vi "Find MFStruct Inner Tunnel.vi"(7 "Source? (T)":bool=TRUE, 8 "error in (no error)":errorcluster, 9 "Tunnel Name":string, 10 "Contained GObject":refnum<vi>, 11 "MFStruct":refnum<vi>) -> (0 "error IO":errorcluster, 1 "Inside Tunnel":refnum<vi>, 2 "GObject dup":refnum<vi>, 3 "MFStruct dup":refnum<vi>)   [LabVIEW 2022 SP3, in "FlexBlocks Support.lvlib"]
uses:
  FlexBlocks Support.lvlib
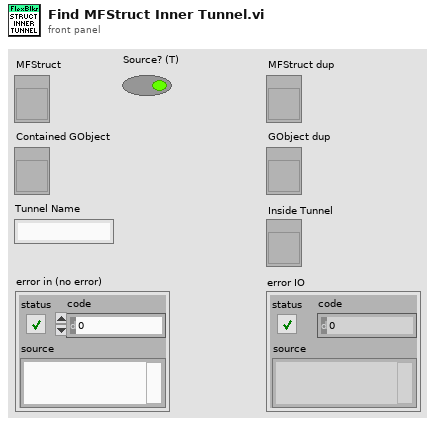
[diagram p1: front panel]
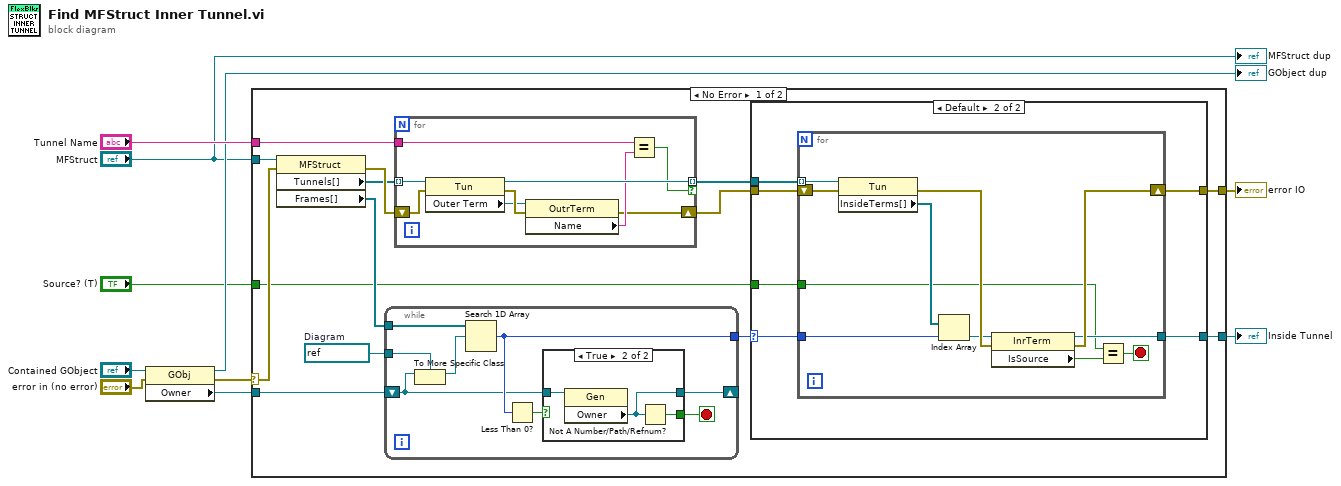
[diagram p0: block diagram]
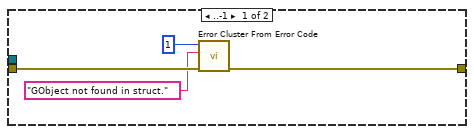
[diagram p2: hidden frame]
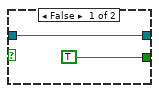
[diagram p3: hidden frame]
diagram:
  n1 = property class="GObj"(reference="Contained GObject", error in="error in (no error)") -> (reference out=→"GObject dup":refnum<vi>, error out=w5:errorcluster, "Owner"=w4:refnum<vi>)
  n2 = case shown="No Error" w5 {
    selector: w5 -> [w20 w68]
    tunnel: "MFStruct" -> [w23 _]
    tunnel: w4 -> [w22 _]
    tunnel: "Tunnel Name" -> [w18 _]
    tunnel: [w16 w68] -> w7
    tunnel: [w13 _] -> w8
    tunnel: "Source? (T)" -> [w11 _]
    frame No Error {
      w12 = refnum<vi> refnum  # Diagram
      n3 = property class="MFStruct"(reference=w23, error in=w20) -> (error out=w24:errorcluster, "Tunnels[]"=w19:refnum<vi>[], "Frames[]"=w21:refnum<vi>[])  [unwired: 1 out]
      n4 = while {
        tunnel: w21 -> [w53]
        tunnel: [w52] -> w14
        shift-right: [w50] -> _
        shift-left: w22 -> [w47]
        tunnel: w12 -> [w49]
        stop <- w46 stop-if-true
        n5 = To More Specific Class(target class=w49, reference=w47) -> (specific class reference=w48:refnum<vi>)  [unwired: 1 in, 1 out]
        n6 = Search 1D Array(1D array=w53, element=w48) -> (index of element=w52:i32)  [unwired: 1 in]
        n7 = Less Than 0?(x=w52) -> (x < 0?=w51:bool)
        n8 = case shown="True" w51 {
          tunnel: w47 -> [w55 w58]
          tunnel: [w55 w57] -> w50
          tunnel: [TRUE w56] -> w46
          frame False {
          }
          frame True {
            n9 = property class="Gen"(reference=w58) -> ("Owner"=w57:refnum<vi>)  [unwired: 1 in, 2 out]
            n10 = Not A Number/Path/Refnum?(number/path/refnum=w57) -> (NaN/Path/Refnum?=w56:bool)
          }
        }
      }
      n11 = for {
        tunnel: w19 -> [w65] mode=indexing
        tunnel: w18 -> [w62]
        tunnel: [w64] -> w15 mode=indexing if=w59
        shift-right: [w60] -> w17
        shift-left: w24 -> [w66]
        n12 = property class="Tun"(reference=w65, error in=w66) -> (reference out=w64:refnum<vi>, error out=w67:errorcluster, "Outer Term"=w63:refnum<vi>)
        n13 = property class="OutrTerm"(reference=w63, error in=w67) -> (error out=w60:errorcluster, "Name"=w61:string)  [unwired: 1 out]
        n14 = Equal?(x=w62, y=w61) -> (x = y?=w59:bool)
      }
      n15 = case shown="Default" w14 {
        selector: w14 -> [_ w31]
        tunnel: w17 -> [w28 w34]
        tunnel: [w27 w33] -> w16
        tunnel: w15 -> [_ w32]
        tunnel: [_ w30] -> w13
        tunnel: w11 -> [_ w29]
        frame ..-1 {
          n16 = call <vilib>:"Error Cluster From Error Code.vi"("error in (no error)"=w28, "error message (\"\")"="GObject not found in struct." ("error message (\"\")"), "error code (0)"=1) -> ("error out"=w27:errorcluster)  [unwired: 6 in]
        }
        frame Default {
          n17 = for {
            tunnel: w32 -> [w43] mode=indexing
            tunnel: w31 -> [w41]
            tunnel: [w38] -> w30
            shift-right: [w45] -> w33
            shift-left: w34 -> [w42]
            tunnel: w29 -> [w36]
            stop <- w35 stop-if-true
            n18 = property class="Tun"(reference=w43, error in=w42) -> (error out=w44:errorcluster, "InsideTerms[]"=w40:refnum<vi>[])  [unwired: 1 out]
            n19 = Index Array(array=w40, index=w41) -> (element=w39:refnum<vi>)
            n20 = property class="InrTerm"(reference=w39, error in=w44) -> (reference out=w38:refnum<vi>, error out=w45:errorcluster, "IsSource"=w37:bool)
            n21 = Equal?(x=w36, y=w37) -> (x = y?=w35:bool)
          }
        }
      }
    }
    frame Error {
    }
  }
  "Inside Tunnel" <- w8
  "error IO" <- w7
  "MFStruct dup" <- "MFStruct"
